vi "GetDaysInMonth.vi"(10 "Year":i32, 11 "Month":i32) -> (2 "Days in Month Array":i32[](array[numeric]), 3 "Number of Days in Month":i32)   [LabVIEW 2015, in "Calendar.lvclass"]
uses:
  Calendar.lvclass
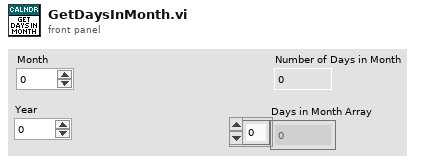
[diagram p1: front panel]
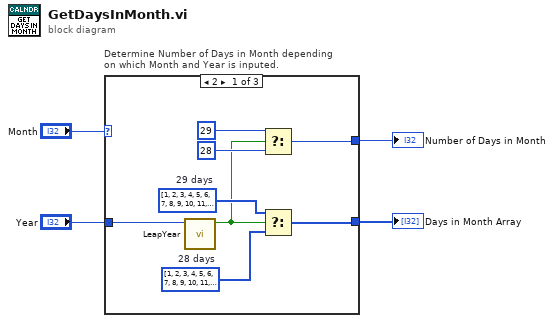
[diagram p0: block diagram]
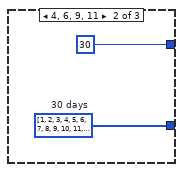
[diagram p2: hidden frame]
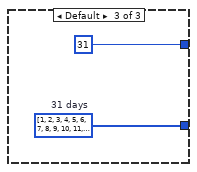
[diagram p3: hidden frame]
diagram:
  n1 = case "Determine Number of Days in Month depending\non which Month and Year is inputed." shown="2" "Month" {
    tunnel: [w12 w14 w16] -> w2
    tunnel: "Year" -> [w6 _ _]
    tunnel: [w7 30 31] -> w1
    frame 2 {
      w11 = i32[] [1, 2, 3, 4, 5, 6, 7, 8, 9, 10, 11, 12, 13, 14, 15, 16, 17, 18, 19, 20, 21, 22, 23, 24, 25, 26, 27, 28]  # 28 days
      w10 = i32[] [1, 2, 3, 4, 5, 6, 7, 8, 9, 10, 11, 12, 13, 14, 15, 16, 17, 18, 19, 20, 21, 22, 23, 24, 25, 26, 27, 28, 29]  # 29 days
      n2 = call "LeapYear.vi"("Year"=w6) -> ("Leap Year?"=w5:bool)  [unwired: 10 in]
      n3 = Select(t=29, s=w5, f=28) -> (s? t:f=w7:i32)
      n4 = Select(t=w10, s=w5, f=w11) -> (s? t:f=w12:i32[])
    }
    frame 4, 6, 9, 11 {
      w14 = i32[] [1, 2, 3, 4, 5, 6, 7, 8, 9, 10, 11, 12, 13, 14, 15, 16, 17, 18, 19, 20, 21, 22, 23, 24, 25, 26, 27, 28, 29, 30]  # 30 days
    }
    frame Default {
      w16 = i32[] [1, 2, 3, 4, 5, 6, 7, 8, 9, 10, 11, 12, 13, 14, 15, 16, 17, 18, 19, 20, 21, 22, 23, 24, 25, 26, 27, 28, 29, 30, 31]  # 31 days
    }
  }
  "Number of Days in Month" <- w1
  "Days in Month Array" <- w2
